vi "Updater Convert TDMS Test Runs 4.3 to 5.0 DC Attenuation.vi"(7 "Source TDMS File In":refnum<k34>, 8 "error in (no error)":errorcluster, 10 "Group Name In":string, 11 "New TDMS File In":refnum<k34>) -> (0 "error out":errorcluster, 2 "Group Name Out":string, 3 "New TDMS File Out":refnum<k34>, 5 "Source TDMS File Out":refnum<k34>)   [LabVIEW 2011]
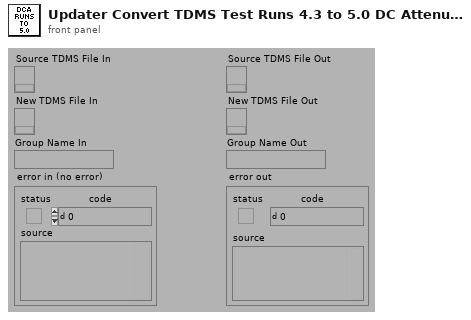
[diagram p1: front panel]
types:
  T1 = typedef "DCA Channel Type.ctl" = enum16{"Data", "Limit", "Invalid", "Topology"}
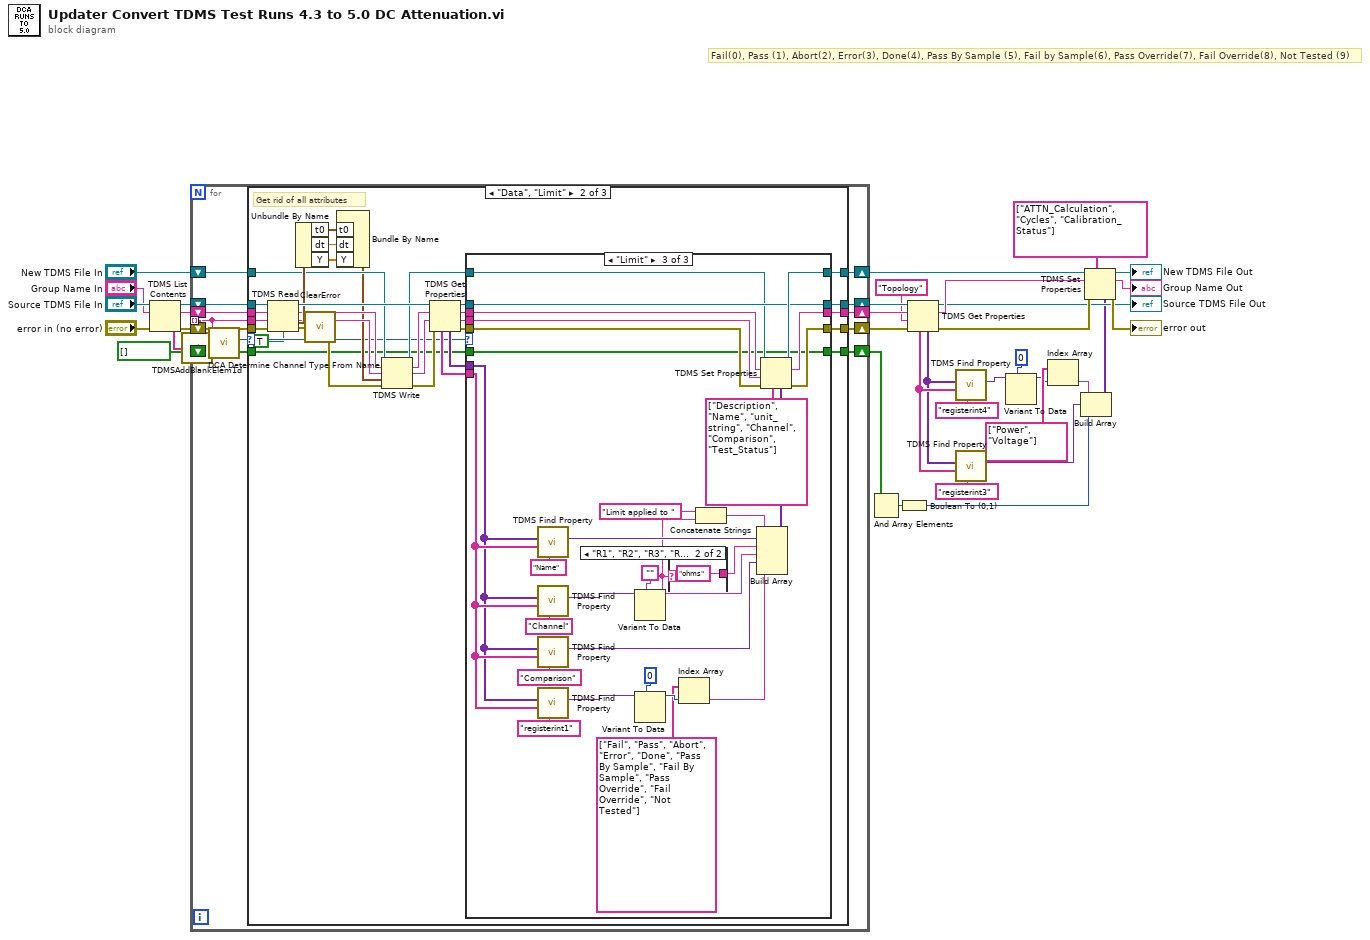
[diagram p0: block diagram]
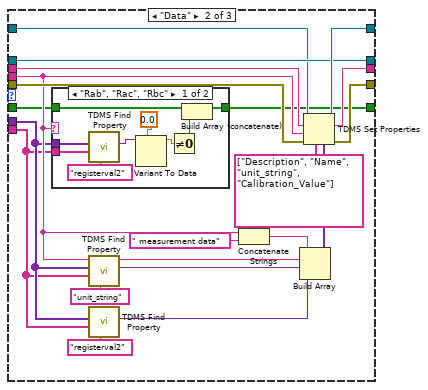
[diagram p4: hidden frame]
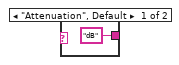
[diagram p6: hidden frame]
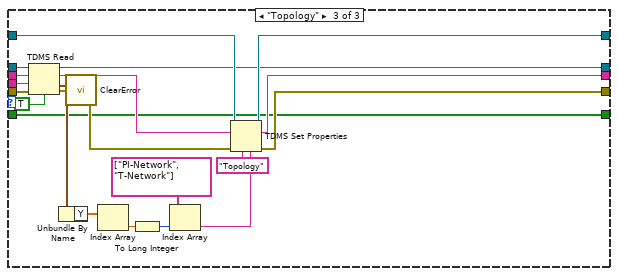
[diagram p7: hidden frame]
diagram:
  # "Fail(0), Pass (1), Abort(2), Error(3), Done(4), Pass By Sample (5), Fail by Sample(6), Pass Override(7), Fail Override(8), Not Tested (9)"
  n1 = TDMS List Contents(4:"error in (no error)", 6:"Group Name In", 7:"Source TDMS File In") -> (0:w33:errorcluster, 1:w1:string[], 2:w31:string, 3:w32:refnum<k34>)
  n2 = call <vilib>:"TDMSAddBlankElem1d.vi"("input string array"=w1) -> ("output string array with blank element at the beginning"=w30:string[])
  n3 = for {
    shift-right: [w47] -> w13
    shift-left: w33 -> [w44]
    shift-right: [w48] -> w29
    shift-left: w32 -> [w43]
    tunnel: w30 -> [w41] mode=indexing
    shift-right: [w46] -> w28
    shift-left: w31 -> [w42]
    shift-right: [w45] -> w20
    shift-left: "New TDMS File In" -> [w40]
    shift-right: [w37] -> w4
    shift-left: bool[] [] -> [w38]
    n4 = call "DCA Determine Channel Type From Name.vi"("Channel Name"=w41) -> ("Channel Type"=w39:T1)  [unwired: 10 out]
    n5 = case shown="\"Data\", \"Limit\"" w39 {
      selector: w39 -> [_ w59 _]
      tunnel: [w53 w86 w163] -> w48
      tunnel: [w50 w85 w164] -> w47
      tunnel: [w52 w84 w162] -> w46
      tunnel: [w51 w83 w174] -> w45
      tunnel: w44 -> [w50 w78 w173]
      tunnel: w43 -> [w53 w76 w172]
      tunnel: w42 -> [w52 w75 w171]
      tunnel: w41 -> [_ w74 w170]
      tunnel: w40 -> [w51 w68 w168]
      tunnel: w38 -> [w49 w57 w156]
      tunnel: [w49 w56 w156] -> w37
      frame "Invalid" {
        # "Empty channel for Group level or Topology"
      }
      frame "Data", "Limit" {
        # "Get rid of all attributes"
        n6 = TDMS Read(0:w76, 5:w75, 7:w74, 11:w78, 13:TRUE ("return channels in file order? (F)")) -> (4:w77:refnum<k34>, 6:w66:string, 8:w65:string, 10:w73:waveform(dbl), 15:w55:errorcluster)  [unwired: 3 in, 1 out]
        n7 = Unbundle By Name(w73) -> ("t0"=w72:timestamp, "dt"=w71:dbl, "Y"=w58:dbl[])
        n8 = call <vilib>:"ClearError.vi"("error in (no error)"=w55) -> ("error out"=w67:errorcluster)
        n9 = Bundle By Name("t0"=w72, "dt"=w71, "Y"=w58) -> (w60:waveform(dbl))  [unwired: 1 out]
        n10 = TDMS Write(0:w68, 5:w66, 7:w65, 9:w60, 11:w67) -> (4:w61:refnum<k34>, 6:w63:string, 8:w64:string, 15:w62:errorcluster)  [unwired: 1 in]
        n11 = TDMS Get Properties(8:w62, 9:w64, 10:w63, 11:w77) -> (0:w82:errorcluster, 1:w81:string, 2:w80:string, 3:w79:refnum<k34>, 4:w69:variant[], 6:w70:string[])  [unwired: 2 out]
        n12 = case shown="\"Limit\"" w59 {
          tunnel: w82 -> [w90 w102 w143]
          tunnel: w80 -> [w89 w106 w146]
          tunnel: w79 -> [w91 w107 w147]
          tunnel: [w91 w107 w147] -> w86
          tunnel: [w90 w109 w149] -> w85
          tunnel: w81 -> [_ w97 w140]
          tunnel: [w89 w110 w150] -> w84
          tunnel: w61 -> [w88 w105 w145]
          tunnel: [w88 w111 w151] -> w83
          tunnel: w70 -> [_ w93 w135]
          tunnel: w69 -> [_ w94 w134]
          tunnel: w57 -> [w87 w96 w123]
          tunnel: [w87 w95 w123] -> w56
          frame Default {
          }
          frame "Data" {
            n13 = case shown="\"Rab\", \"Rac\", \"Rbc\"" w97 {
              tunnel: w96 -> [w120 w121]
              tunnel: [w119 w121] -> w95
              tunnel: w94 -> [w113 _]
              tunnel: w93 -> [w112 _]
              frame "Rab", "Rac", "Rbc" {
                n14 = call "TDMS Find Property.vi"("Property Name"="registerval2", "Property Names"=w112, "Property Values"=w113) -> ("Property Value"=w115:variant)  [unwired: 5 out]
                n15 = Variant To Data(type=0.0, Variant=w115) -> (data=w114:dbl)  [unwired: 1 in, 1 out]
                n16 = Not Equal To 0?(x=w114) -> (x != 0?=w118:bool)
                n17 = Build Array (concatenate)(w120, w118) -> (w119:bool[])
              }
              frame Default {
              }
            }
            n18 = call "TDMS Find Property.vi"("Property Name"="unit_string", "Property Names"=w93, "Property Values"=w94) -> ("Property Value"=w98:variant)  [unwired: 5 out]
            n19 = call "TDMS Find Property.vi"("Property Name"="registerval2", "Property Names"=w93, "Property Values"=w94) -> ("Property Value"=w100:variant)  [unwired: 5 out]
            n20 = Concatenate Strings(w97, " measurement data" ("string")) -> (w92:string)
            n21 = Build Array(w92, w97, w98, w100) -> (w101:variant[])
            n22 = TDMS Set Properties(5:w101, 7:string[] ["Description", "Name", "unit_string", "Calibration_Value"], 8:w102, 9:w97, 10:w106, 11:w105) -> (0:w109:errorcluster, 2:w110:string, 3:w111:refnum<k34>)  [unwired: 1 out]
          }
          frame "Limit" {
            n23 = call "TDMS Find Property.vi"("Property Name"="Name", "Property Names"=w135, "Property Values"=w134) -> ("Property Value"=w138:variant)  [unwired: 5 out]
            n24 = call "TDMS Find Property.vi"("Property Name"="Channel", "Property Names"=w135, "Property Values"=w134) -> ("Property Value"=w126:variant)  [unwired: 5 out]
            n25 = call "TDMS Find Property.vi"("Property Name"="Comparison", "Property Names"=w135, "Property Values"=w134) -> ("Property Value"=w128:variant)  [unwired: 5 out]
            n26 = call "TDMS Find Property.vi"("Property Name"="registerint1", "Property Names"=w135, "Property Values"=w134) -> ("Property Value"=w132:variant)  [unwired: 5 out]
            n27 = Variant To Data(type="", Variant=w126) -> (data=w124:string)  [unwired: 1 in, 1 out]
            n28 = Variant To Data(type=0, Variant=w132) -> (data=w131:i32)  [unwired: 1 in, 1 out]
            n29 = case shown="\"R1\", \"R2\", \"R3\", \"Rab\", \"Rac\", \"Rbc\", \"Zin\", \"Zo\", \"Zout\"" w124 {
              tunnel: ["dB" "ohms"] -> w125
              frame "Attenuation", Default {
              }
              frame "R1", "R2", "R3", "Rab", "Rac", "Rbc", "Zin", "Zo", "Zout" {
              }
            }
            n30 = Index Array(array=string[] ["Fail", "Pass", "Abort", "Error", "Done", "Pass By Sample", "Fail By Sample", "Pass Override", "Fail Override", "Not Tested"], index=w131) -> (element=w129:string)
            n31 = Concatenate Strings("Limit applied to " ("string"), w124) -> (w122:string)
            n32 = Build Array(w122, w138, w125, w124, w128, w129) -> (w142:variant[])
            n33 = TDMS Set Properties(5:w142, 7:string[] ["Description", "Name", "unit_string", "Channel", "Comparison", "Test_Status"], 8:w143, 9:w140, 10:w146, 11:w145) -> (0:w149:errorcluster, 2:w150:string, 3:w151:refnum<k34>)  [unwired: 1 out]
          }
        }
      }
      frame "Topology" {
        n34 = TDMS Read(0:w172, 5:w171, 7:w170, 11:w173, 13:TRUE ("return channels in file order? (F)")) -> (4:w163:refnum<k34>, 6:w166:string, 10:w169:waveform(dbl), 15:w155:errorcluster)  [unwired: 3 in, 2 out]
        n35 = Unbundle By Name(w169) -> ("Y"=w165:dbl[])
        n36 = call <vilib>:"ClearError.vi"("error in (no error)"=w155) -> ("error out"=w167:errorcluster)
        n37 = Index Array(array=w165) -> (element=w161:dbl)  [unwired: 1 in]
        n38 = To Long Integer(number=w161) -> (32bit integer=w160:i32)
        n39 = Index Array(array=string[] ["PI-Network", "T-Network"], index=w160) -> (element=w158:string)
        n40 = TDMS Set Properties(5:w158, 7:"Topology" ("property names"), 8:w167, 10:w166, 11:w168) -> (0:w164:errorcluster, 2:w162:string, 3:w174:refnum<k34>)  [unwired: 2 out]
      }
    }
  }
  n41 = And Array Elements(Boolean array=w4) -> (logical AND=w3:bool)
  n42 = Boolean To (0,1)(Boolean=w3) -> (0, 1=w2:i16)
  n43 = TDMS Get Properties(8:w13, 9:"Topology", 10:w28, 11:w29) -> (0:w27:errorcluster, 2:w25:string, 3:→"Source TDMS File Out":refnum<k34>, 4:w10:variant[], 6:w11:string[])  [unwired: 1 in, 2 out]
  n44 = call "TDMS Find Property.vi"("Property Name"="registerint4", "Property Names"=w11, "Property Values"=w10) -> ("Property Value"=w17:variant)  [unwired: 5 out]
  n45 = call "TDMS Find Property.vi"("Property Name"="registerint3", "Property Names"=w11, "Property Values"=w10) -> ("Property Value"=w8:variant)  [unwired: 5 out]
  n46 = Variant To Data(type=0, Variant=w17) -> (data=w14:i32)  [unwired: 1 in, 1 out]
  n47 = Index Array(array=string[] ["Power", "Voltage"], index=w14) -> (element=w7:string)
  n48 = Build Array(w7, w8, w2) -> (w6:variant[])
  n49 = TDMS Set Properties(5:w6, 7:string[] ["ATTN_Calculation", "Cycles", "Calibration_Status"], 8:w27, 10:w25, 11:w20) -> (0:→"error out":errorcluster, 2:→"Group Name Out":string, 3:→"New TDMS File Out":refnum<k34>)  [unwired: 2 out]
